vi "SavePointables.vi"(10 "error in (no error)":errorcluster, 11 "Leap Pointables":refnum<k24>) -> (2 "error out":errorcluster, 3 "Pointables":T1[](array[typedef]))   [LabVIEW 2011, in "LVH-Leap.lvlib"]
uses:
  LVH-Leap.lvlib
  Type Defs/Pointable.ctl
  Type Defs/Pointable Type.ctl
  Type Defs/Pointable Zone.ctl
  Type Defs/Vector.ctl
  C:/github/labviewhacker/LVH-Leap/LabVIEW/vi.lib/LabVIEW Hacker/Leap/Private/Libs/LeapCSharp.NET3.5.dll
  Libs/LeapCSharp.NET3.5.dll
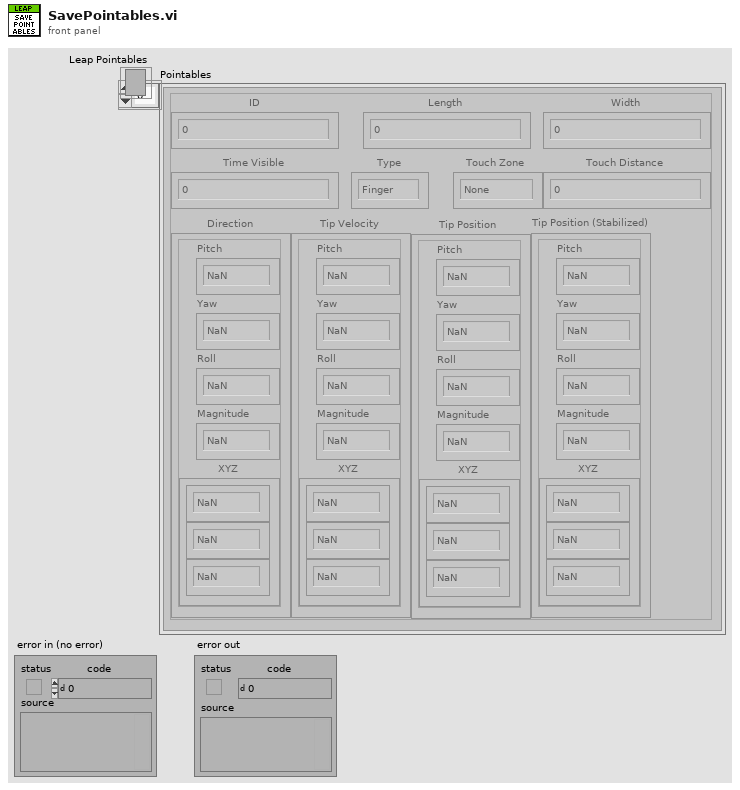
[diagram p1: front panel]
types:
  T1 = typedef "LVH-Leap.lvlib/Pointable.ctl" = cluster{"Type":T2, "Touch Zone":T3, "ID":i32, "Length":dbl, "Width":dbl, "Time Visible":dbl, "Touch Distance":dbl, "Direction":T4, "Tip Position":T4, "Tip Velocity":T4, "Tip Position (Stabilized)":T4}
  T2 = typedef "LVH-Leap.lvlib/Pointable Type.ctl" = enum16{"Finger", "Tool"}
  T3 = typedef "LVH-Leap.lvlib/Pointable Zone.ctl" = enum16{"None", "Hovering", "Touching"}
  T4 = typedef "LVH-Leap.lvlib/Vector.ctl" = cluster{"Pitch":sgl, "Yaw":sgl, "Roll":sgl, "Magnitude":sgl, "XYZ":sgl[]}
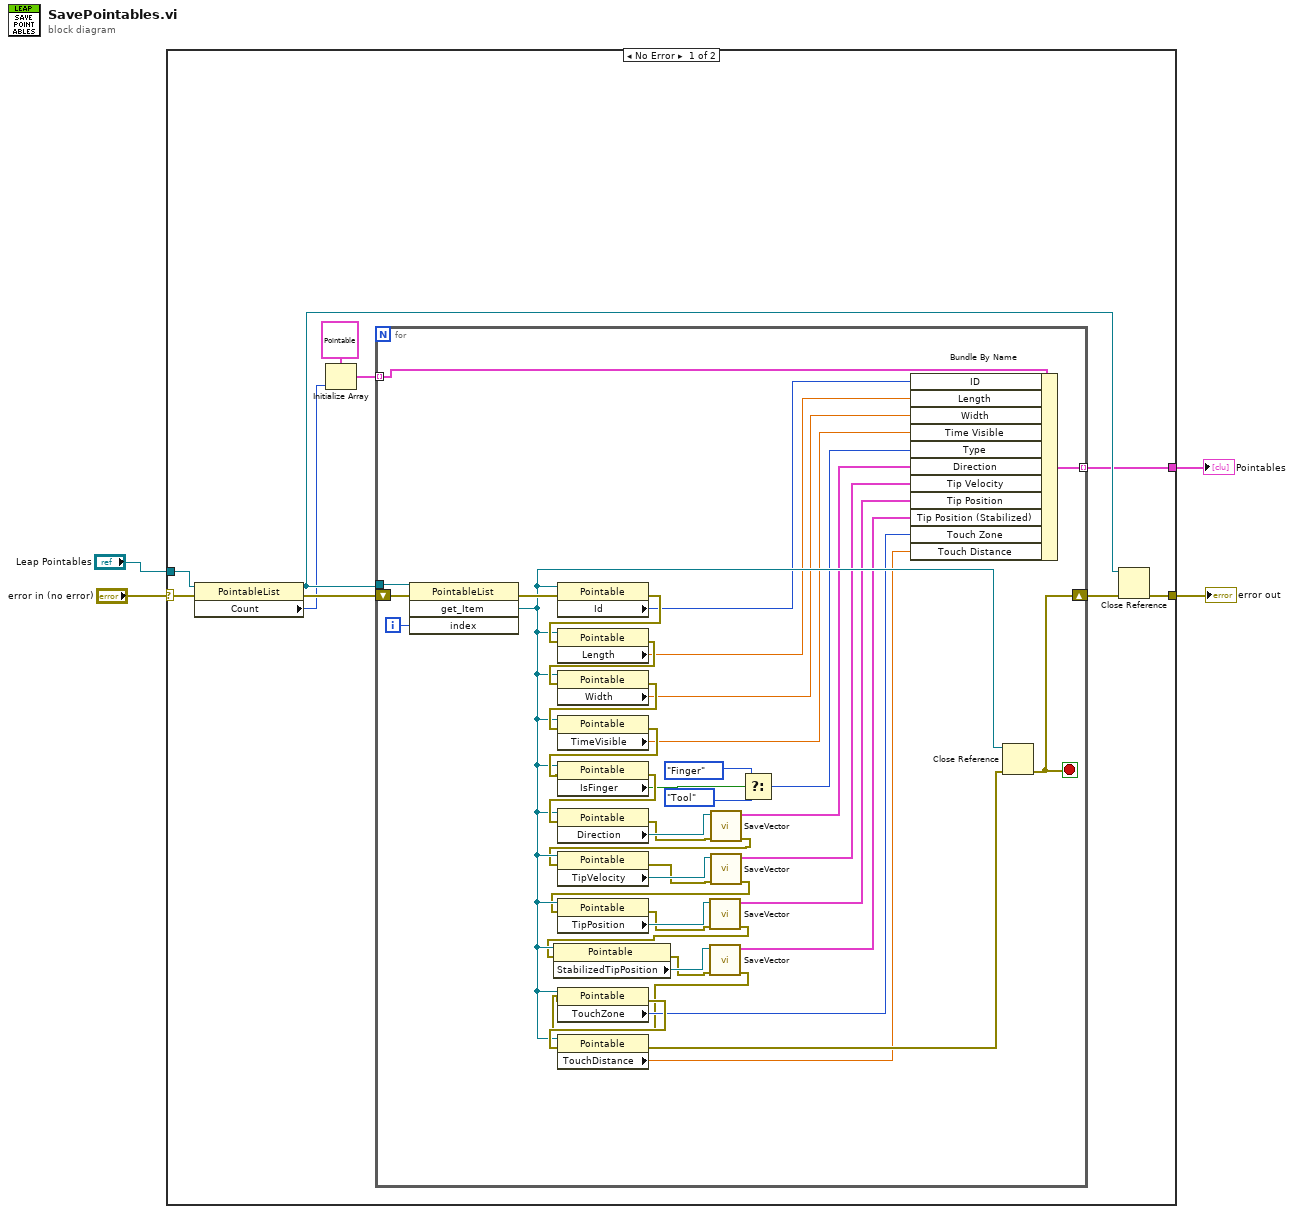
[diagram p0: block diagram]
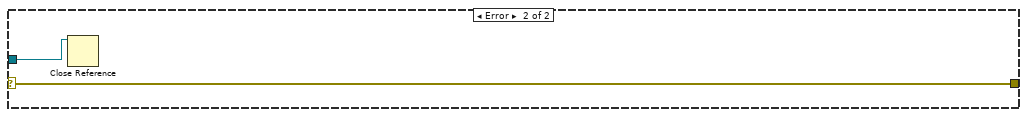
[diagram p2: hidden frame]
diagram:
  n1 = case shown="No Error" "error in (no error)" {
    selector: "error in (no error)" -> [w8 w57]
    tunnel: [w12 _] -> w2
    tunnel: "Leap Pointables" -> [w9 w56]
    tunnel: [w6 w57] -> w3
    frame No Error {
      n2 = property class="PointableList"(reference=w9, error in=w8) -> (reference out=w13:refnum<k24>, error out=w14:errorcluster, "Count"=w10:i32)
      n3 = Initialize Array(T1 {"Type"=enum."Finger", "Touch Zone"=enum."None", "ID"=0, "Length"=0.0, "Width"=0.0, "Time Visible"=0.0, "Touch Distance"=0.0, "Direction"={"Pitch"=0.0, "Yaw"=0.0, "Roll"=0.0, "Magnitude"=0.0, "XYZ"=[]}, "Tip Position"={"Pitch"=0.0, "Yaw"=0.0, "Roll"=0.0, "Magnitude"=0.0, "XYZ"=[]}, "Tip Velocity"={"Pitch"=0.0, "Yaw"=0.0, "Roll"=0.0, "Magnitude"=0.0, "XYZ"=[]}, "Tip Position (Stabilized)"={"Pitch"=0.0, "Yaw"=0.0, "Roll"=0.0, "Magnitude"=0.0, "XYZ"=[]}} ("Finger"), w10) -> (w11:T1[])
      n4 = for {
        tunnel: w13 -> [w46]
        tunnel: w11 -> [w44] mode=indexing
        tunnel: [w43] -> w12 mode=indexing
        shift-right: [w36] -> w7
        shift-left: w14 -> [w47]
        i -> [w45]
        stop <- w36 stop-if-true
        n5 = invoke class="PointableList" method="get_Item"(reference=w46, error in=w47, "index"=w45) -> (error out=w55:errorcluster, "get_Item"=w48:refnum<k24>)  [unwired: 1 in, 2 out]
        n6 = property class="Pointable"(reference=w48, error in=w55) -> (error out=w49:errorcluster, "Id"=w37:i32)  [unwired: 1 out]
        n7 = property class="Pointable"(reference=w48, error in=w49) -> (error out=w50:errorcluster, "Length"=w38:sgl)  [unwired: 1 out]
        n8 = property class="Pointable"(reference=w48, error in=w50) -> (error out=w51:errorcluster, "Width"=w39:sgl)  [unwired: 1 out]
        n9 = property class="Pointable"(reference=w48, error in=w51) -> (error out=w52:errorcluster, "TimeVisible"=w30:sgl)  [unwired: 1 out]
        n10 = property class="Pointable"(reference=w48, error in=w52) -> (error out=w53:errorcluster, "IsFinger"=w34:bool)  [unwired: 1 out]
        n11 = property class="Pointable"(reference=w48, error in=w53) -> (error out=w23:errorcluster, "Direction"=w40:refnum<k24>)  [unwired: 1 out]
        n12 = call "SaveVector.vi"("error in (no error)"=w23, "Leap Vector"=w40) -> ("error out"=w22:errorcluster, "Vector"=w28:T4)  [unwired: 8 in]
        n13 = property class="Pointable"(reference=w48, error in=w22) -> (error out=w21:errorcluster, "TipVelocity"=w41:refnum<k24>)  [unwired: 1 out]
        n14 = call "SaveVector.vi"("error in (no error)"=w21, "Leap Vector"=w41) -> ("error out"=w19:errorcluster, "Vector"=w27:T4)  [unwired: 8 in]
        n15 = property class="Pointable"(reference=w48, error in=w19) -> (error out=w18:errorcluster, "TipPosition"=w42:refnum<k24>)  [unwired: 1 out]
        n16 = call "SaveVector.vi"("error in (no error)"=w18, "Leap Vector"=w42) -> ("error out"=w17:errorcluster, "Vector"=w26:T4)  [unwired: 8 in]
        n17 = property class="Pointable"(reference=w48, error in=w17) -> (error out=w16:errorcluster, "StabilizedTipPosition"=w35:refnum<k24>)  [unwired: 1 out]
        n18 = call "SaveVector.vi"("error in (no error)"=w16, "Leap Vector"=w35) -> ("error out"=w15:errorcluster, "Vector"=w25:T4)  [unwired: 8 in]
        n19 = property class="Pointable"(reference=w48, error in=w15) -> (error out=w54:errorcluster, "TouchZone"=w24:i32)  [unwired: 1 out]
        n20 = property class="Pointable"(reference=w48, error in=w54) -> (error out=w31:errorcluster, "TouchDistance"=w20:sgl)  [unwired: 1 out]
        n21 = Select(t=Pointable_Type."Finger" ("pointable type"), s=w34, f=Pointable_Type."Tool" ("pointable type")) -> (s? t:f=w29:T2)
        n22 = Bundle By Name(cluster=w44, "ID"=w37, "Length"=w38, "Width"=w39, "Time Visible"=w30, "Type"=w29, "Direction"=w28, "Tip Velocity"=w27, "Tip Position"=w26, "Tip Position (Stabilized)"=w25, "Touch Zone"=w24, "Touch Distance"=w20) -> (w43:T1)
        n23 = Close Reference(reference=w48, error in (no error)=w31) -> (error out=w36:errorcluster)
      }
      n24 = Close Reference(reference=w13, error in (no error)=w7) -> (error out=w6:errorcluster)
    }
    frame Error {
      n25 = Close Reference(reference=w56) -> ()  [unwired: 1 in, 1 out]
    }
  }
  "Pointables" <- w2
  "error out" <- w3
